vi "libssh2_sftp_symlink.vi"(8 "error in (no error)":errorcluster, 9 "target":string, 10 "path":string, 11 "sftp":T1) -> (0 "error out":errorcluster)   [LabVIEW 2013, in "libssh2.lvlib"]
doc: "Create a symbolic link."
uses:
  libssh2.lvlib
  SFTP Refnum.ctl
  libssh2_sftp_symlink_type.ctl
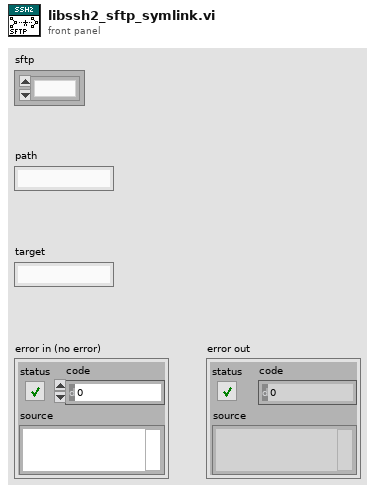
[diagram p1: front panel]
types:
  T1 = typedef "libssh2.lvlib/SFTP Refnum.ctl" = refnum<k1>
  T2 = typedef "libssh2.lvlib/libssh2_sftp_symlink_type.ctl" = enum16{"SYMLINK", "READLINK", "REALPATH"}
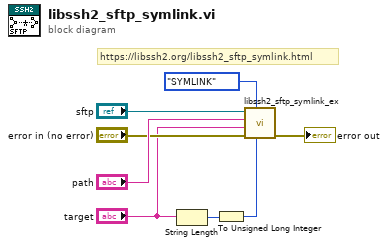
[diagram p0: block diagram]
diagram:
  # "https://libssh2.org/libssh2_sftp_symlink.html"
  n1 = String Length(string="target") -> (length=w2:i32)
  n2 = To Unsigned Long Integer(number=w2) -> (unsigned 32bit integer=w1:u32)
  n3 = call "libssh2_sftp_symlink_ex.vi"("target_len"=w1, "link_type"=libssh2_sftp_symlink_type."SYMLINK" ("link type"), "error in (no error)"="error in (no error)", "target in"="target", "path"="path", "sftp"="sftp") -> ("error out"=→"error out":errorcluster)  [unwired: 4 in, 1 out]
